vi "Create Pattern Script(Addr_3W).vi"(8 "error in (no error)":errorcluster, 11 "Addr":u16 format="%x") -> (0 "error out":errorcluster, 3 "String":string)   [LabVIEW 2018, in "SPI_Frame_Root.lvclass"]
uses:
  SPI_Frame_Root.lvclass
  Classes/BML_Frame_Root/BML_Frame_Root.lvclass
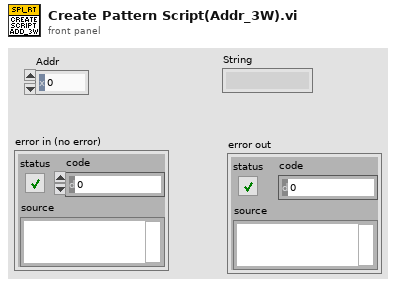
[diagram p1: front panel]
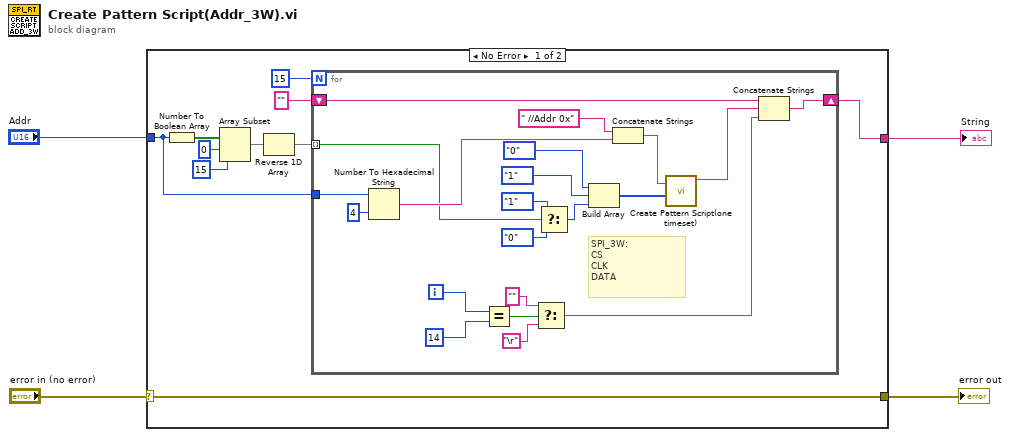
[diagram p0: block diagram]
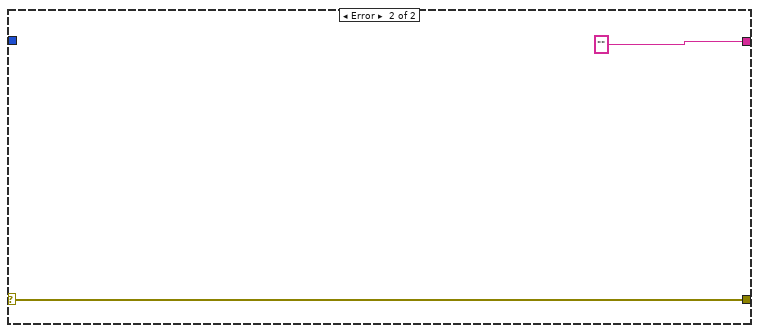
[diagram p2: hidden frame]
diagram:
  n1 = case shown="No Error" "error in (no error)" {
    selector: "error in (no error)" -> [w14 w36]
    tunnel: [w11 ""] -> w3
    tunnel: [w14 w36] -> w2
    tunnel: "Addr" -> [w10 _]
    frame No Error {
      n2 = Number To Boolean Array(number=w10) -> (Boolean array=w9:bool[])
      n3 = Array Subset(array=w9, index=0, length=15) -> (w6:bool[])
      n4 = Reverse 1D Array(array=w6) -> (reversed array=w5:bool[])
      n5 = for {
        N: 15 -> [_]
        shift-right: [w30] -> w11
        shift-left: "" -> [w29]
        tunnel: w10 -> [w28]
        tunnel: w5 -> [w19] mode=indexing
        i -> [w20]
        # "SPI_3W:\nCS\nCLK\nDATA"
        n6 = Number To Hexadecimal String(1:i16 4 ("width (-)"), 2:w28) -> (0:w26:string)
        n7 = Equal?(x=w20, y=14) -> (x = y?=w34:bool)
        n8 = Select(t="", s=w34, f="\r") -> (s? t:f=w31:string)
        n9 = Select(t=enum16{"0", "1", "L", "H", "X", "V", "D", "M"}."1" ("PinState"), s=w19, f=enum16{"0", "1", "L", "H", "X", "V", "D", "M"}."0") -> (s? t:f=w16:enum16{"0", "1", "L", "H", "X", "V", "D", "M"})
        n10 = Build Array(enum16{"0", "1", "L", "H", "X", "V", "D", "M"}."0" ("element"), enum16{"0", "1", "L", "H", "X", "V", "D", "M"}."1" ("element"), w16) -> (w24:enum16{"0", "1", "L", "H", "X", "V", "D", "M"}[])
        n11 = Concatenate Strings(" //Addr 0x" ("Notes"), w26) -> (w21:string)
        n12 = call "Create Pattern Script(one timeset).vi"("Notes"=w21, "PinState"=w24) -> ("string out"=w18:string)  [unwired: 9 in]
        n13 = Concatenate Strings(w29, w18, w31) -> (w30:string)
      }
    }
    frame Error {
    }
  }
  "String" <- w3
  "error out" <- w2
